vi "Convert Callback To Selected Item.vi"(8 "error in":errorcluster, 11 "Data":variant) -> (0 "error out":errorcluster, 3 "Selected Item":T1)   [LabVIEW 2020, in "NI_VS UI Single Node Browser.lvlib"]
uses:
  <vilib>/NI VeriStand/UI Controls/Single Node Browser/NI_VS UI Single Node Browser.lvlib
  <vilib>/NI VeriStand/UI Controls/Single Node Browser/Node Ref.ctl
  NationalInstruments.VeriStand.SystemStorage
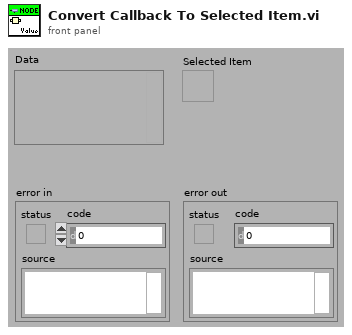
[diagram p1: front panel]
types:
  T1 = typedef "NI_VS UI Single Node Browser.lvlib/Node Ref.ctl" = refnum<k24>
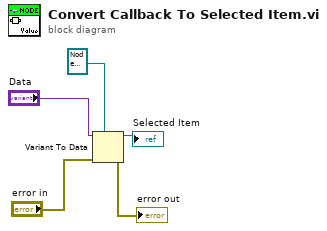
[diagram p0: block diagram]
diagram:
  n1 = Variant To Data(error in="error in", type=T1 refnum ("Selected Item"), Variant="Data") -> (data=→"Selected Item":T1, error out=→"error out":errorcluster)
